vi "Write G08_Chnl_Settings.vi"(8 "error in (no error)":errorcluster, 10 "G08_Chnl_Settings":T1={"Pulse Width (µs)"=0.005, "Output Offset"=0, "Disconnect (E,F)"=FALSE, "Onto MsBus (E,F)"=FALSE, "Input Positive (E,F)"=TRUE} {"Pulse Width (µs)" min=0.0 max=8947840.0 format="%#.6f"}, 11 "BME_DG_G08_Chnl in":refnum<class "BME_DG_G08_Chnl.lvclass">) -> (0 "error out":errorcluster, 3 "BME_DG_G08_Chnl out":refnum<class "BME_DG_G08_Chnl.lvclass">)   [LabVIEW 2009, in "POLARIS BME DG.lvlib" / "BME_DG_G08_Chnl.lvclass"]
uses:
  BME_DG_G08_Chnl.lvclass
  LV-BME Interface/SG08_Chnl_Settings.ctl
  BME_DG_G08_Chnl.lvclass/BME_DG_G08_Chnl.ctl
  POLARIS BME DG.lvlib
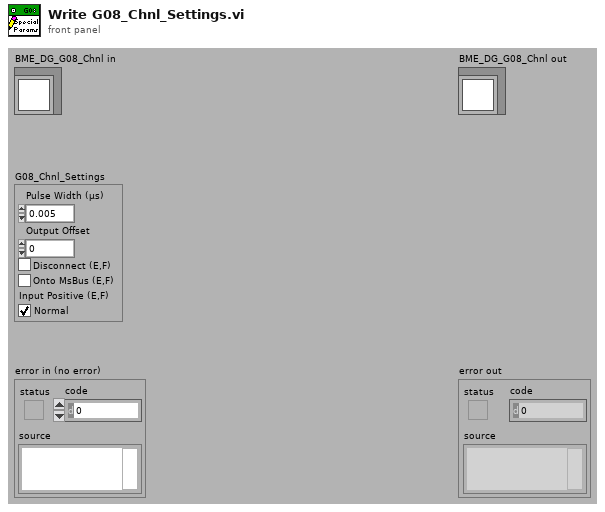
[diagram p1: front panel]
types:
  T1 = typedef "POLARIS BME DG.lvlib/SG08_Chnl_Settings.ctl" = cluster{"Pulse Width (µs)":dbl, "Output Offset":u32, "Disconnect (E,F)":bool, "Onto MsBus (E,F)":bool, "Input Positive (E,F)":bool}
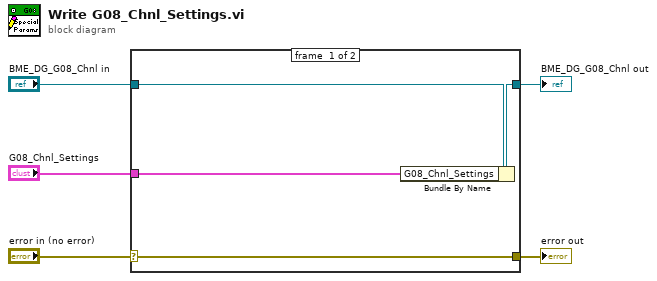
[diagram p0: block diagram]
diagram:
  n1 = case shown="No Error" "error in (no error)" {
    selector: "error in (no error)" -> [w9 w10]
    tunnel: [w9 w10] -> w4
    tunnel: [w7 w11] -> w2
    tunnel: "BME_DG_G08_Chnl in" -> [w8 w11]
    tunnel: "G08_Chnl_Settings" -> [w6 _]
    frame #0 {
      n2 = Bundle By Name(cluster=w8, "G08_Chnl_Settings"=w6) -> (w7:refnum<class "BME_DG_G08_Chnl.lvclass">)
    }
    frame #1 {
    }
  }
  "error out" <- w4
  "BME_DG_G08_Chnl out" <- w2
